vi "[TEST] A3200 Control.vi"() -> ()   [LabVIEW 2026]
uses:
  <extravilib>/ChannelInstances/Tag-str/Write With Abort.vi
  <extravilib>/ChannelInstances/Tag-str/Read With Abort.vi
  <extravilib>/ChannelInstances/Tag-str/Instantiate.vi
  <extravilib>/ChannelInstances/Tag-str/EndpointRead.vi
  <instrlib>/A3200/Motion/AbortSingle.vi
  <instrlib>/A3200/Motion/DisableSingle.vi
  <instrlib>/A3200/Motion/EnableSingle.vi
  <instrlib>/A3200/Motion/FreerunSingle.vi
  <extravilib>/ChannelInstances/Tag-str/Endpoint.vi
  <instrlib>/A3200/Parameters/GetAxisParameterString.vi
  <instrlib>/A3200/Parameters/GetAxisParameterDouble.vi
  <extravilib>/ChannelInstances/Tag-str.lvlib
panel:
  in  "Cluster":T1
  in  "Disable Axis":bool
  in  "ACK ALL":bool
  in  "Enable Axis":bool
  out "Velocity Feedback":string
  out "Position Fbk":string
  out "Numeric":dbl format="%#_13g"
  in  "Stop 3":bool
  in  "Axis Select":i32
  in  "Distance":dbl=1000.0 min=0.0 max=2000.0
  in  "Speed":dbl=5000.0 min=0.0 max=50.0
  out "Status":string
  out "Vel Fbk":dbl
  out "Pos Units":string
  out "Vel Units":string
  in  "Disconnect?":bool
  in  "Stop 2":bool
  out "Axis Selected":string
  in  "Stop":bool
  in  "Go To":bool
  in  "Right":bool
  in  "Left":bool
  out "Encoder X Value":dbl
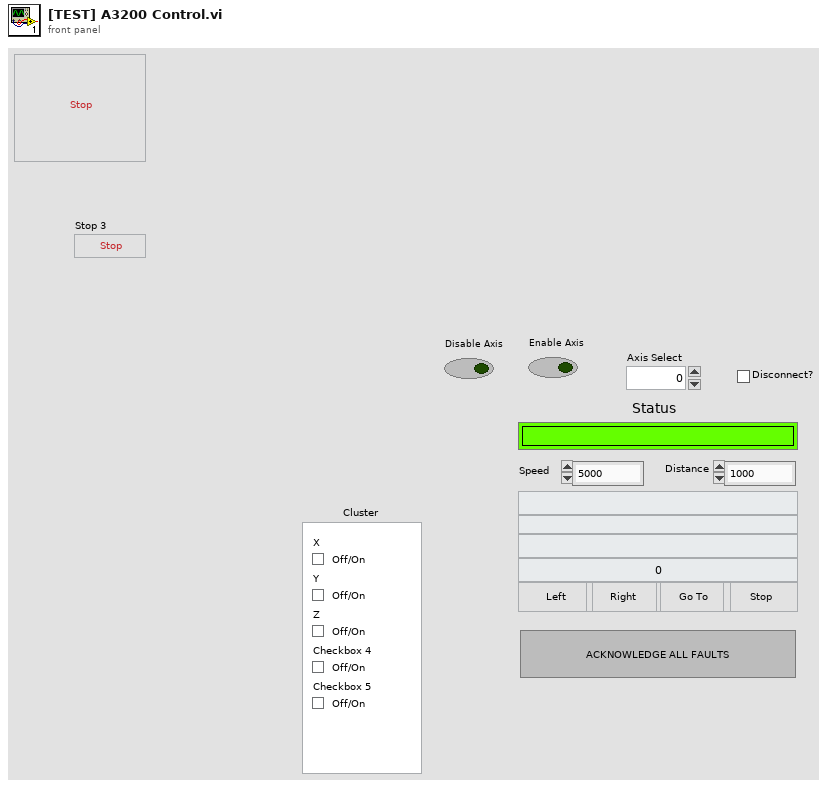
[diagram p1: front panel]
types:
  T1 = cluster{"X":bool, "Y":bool, "Z":bool, "Checkbox 4":bool, "Checkbox 5":bool}
  T2 = cluster{"new reference":refnum<k24>, "Event Callback":refnum<k27>, "ControllerDiagPacket":refnum<user-event>, "Event Registration Refnum":refnum<event-registration>}
  T3 = typedef "AxisDiagPacket.ctl" = cluster{"Axis Name":string, "Analog Input 0":dbl, "Analog Input 1":dbl, "Axis Fault (num)":i32, "Axis Fault (str)":string, "Axis Fault (bits)":cluster{"AmplifierFault":bool, "AmplifierTemperatureFault":bool, "CcwEndOfTravelLimitFault":bool, "CcwSoftwareLimitFault":bool, "CommunicationLostFault":bool, "CwEndOfTravelLimitFault":bool, "CwSoftwareLimitFault":bool, "EmergencyStopFault":bool, "EncoderFault":bool, "ExternalFault":bool, "FeedbackScalingFault":bool, "GantryMisalignFault ":bool, "HallSensorFault":bool, "InPositionTimeoutFault":bool, "MarkerSearchFault":bool, "MaxVelocityCommandFault":bool, "MissedInterruptFault":bool, "MotorTemperatureFault":bool, "None":bool, "OverCurrentFault":bool, "PositionErrorFault":bool, "PositionFeedbackFault":bool, "PowerSupplyFault":bool, "ProbeInputFault":bool, "SafeZoneFault":bool, "VelocityErrorFault":bool, "VelocityFeedbackFault":bool, "VoltageClampFault":bool, "InternalFault":bool}, "Axis Status (num)":i32, "Axis Status (str)":string, "Axis Status (bits)":cluster{"BacklashActive":bool, "CalibrationEnabled1D":bool, "CalibrationEnabled2D":bool, "CommandValid":bool, "DriveAbortPending":bool, "DrivePending":bool, "Enabling":bool, "GainMappingEnabled":bool, "GantryAligned":bool, "GantryRealigning":bool, "Homed":bool, "Homing":bool, "IFOVEnabled":bool, "JogGenerating":bool, "Jogging":bool, "JoystickControl":bool, "MasterSlaveControl":bool, "MotionBlocked":bool, "MotionClamped":bool, "MoveDone":bool, "None":bool, "NotVirtual":bool, "Profiling":bool, "Stability0":bool, "Stability1":bool, "TrajectoryFiltering":bool, "WaitDone":bool}, "Current Command":sgl, "Current Error":sgl, "Current Feedback":sgl, "Digital Inputs":i32, "Digital Outputs":i32, "Drive Status":i32, "Drive Status (str)":string, "Drive Status (bits)":cluster{"AccelerationPhase":bool, "AutofocusActive":bool, "BrakeOutput":bool, "CcwEndOfTravelLimitInput":bool, "CosineEncoderError":bool, "CurrentClamp":bool, "CwEndOfTravelLimitInput":bool, "DecelerationPhase":bool, "DualLoopActive":bool, "EmergencyStopInput":bool, "Enabled":bool, "EncoderClipping":bool, "GalvoCalibrationEnabled":bool, "GalvoPowerCorrection":bool, "HallAInput":bool, "HallBInput":bool, "HallCInput":bool, "HighResolutionMode":bool, "HomeLimitInput":bool, "InPosition":bool, "InPosition2":bool, "MarkerInput":bool, "MarkerLatch":bool, "MoveActive":bool, "NoMotorSupply":bool, "None":bool, "PowerLimiting":bool, "ProgrammingFlash":bool, "ProgrammingMXH":bool, "PSOHaltLatch":bool, "ServoControl":bool, "SineEncoderError":bool}, "Position Feedback Auxiliary":dbl, "Position Command":dbl, "Position Error":dbl, "Position Feedback":dbl, "Program Position Command":dbl, "Program Position Error":dbl, "Program Position Feedback":dbl, "Velocity Command":dbl, "Velocity Error":dbl, "Velocity Feedback":dbl}
  T4 = typedef "Tag-str.lvlib/))Channel.ctl" = refnum<queue>
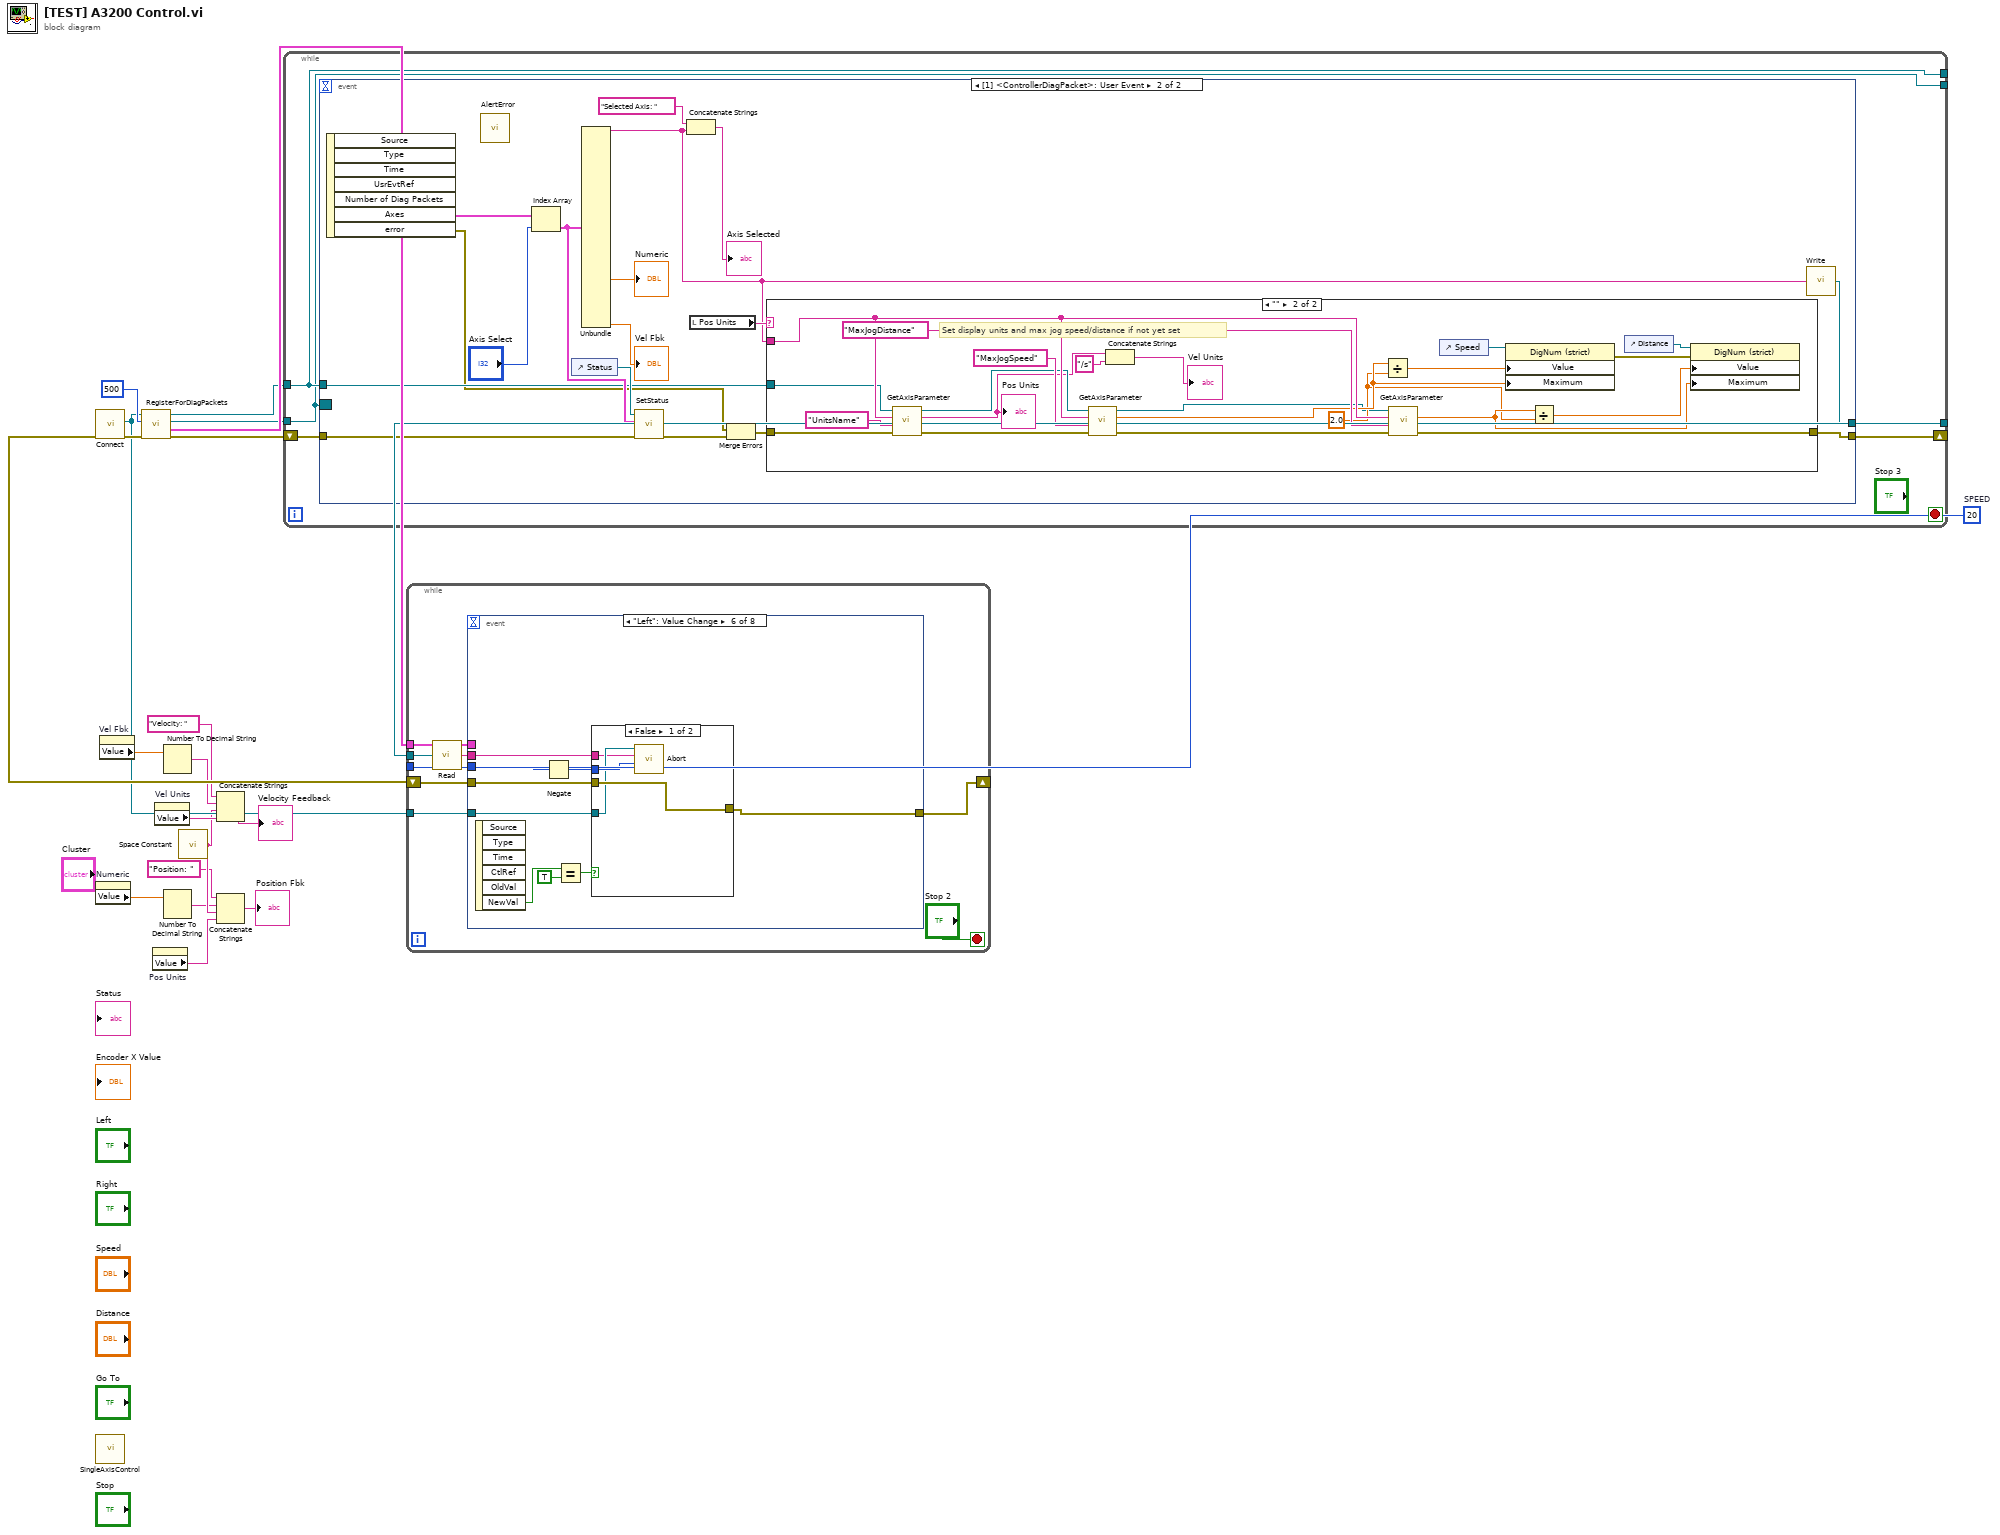
[diagram p0: block diagram]
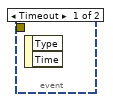
[diagram p2: hidden frame]
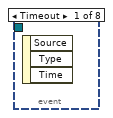
[diagram p4: hidden frame]
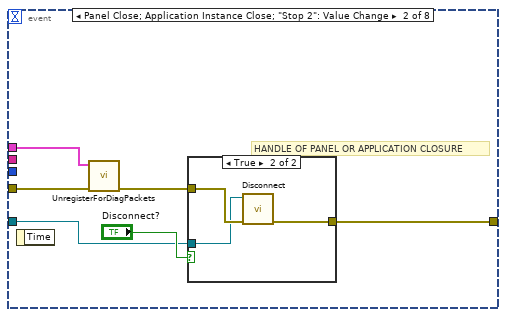
[diagram p5: hidden frame]
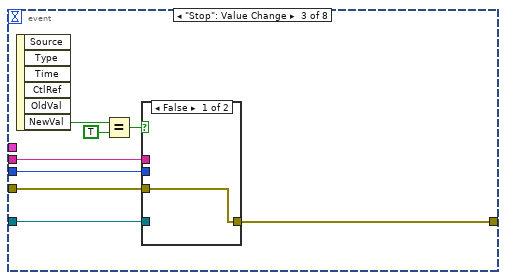
[diagram p7: hidden frame]
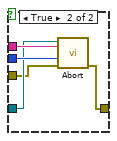
[diagram p8: hidden frame]
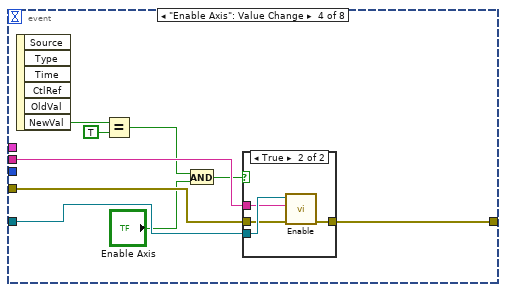
[diagram p9: hidden frame]
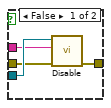
[diagram p10: hidden frame]
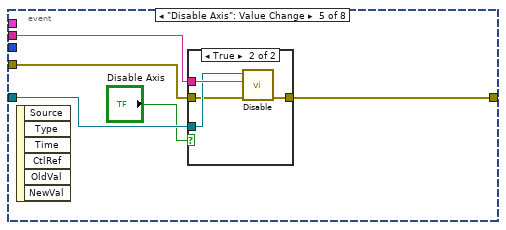
[diagram p11: hidden frame]
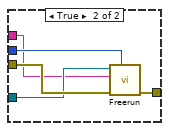
[diagram p13: hidden frame]
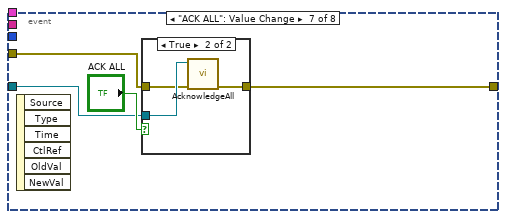
[diagram p14: hidden frame]
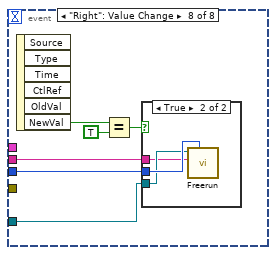
[diagram p16: hidden frame]
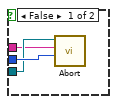
[diagram p17: hidden frame]
diagram:
  w20 = 20  # SPEED
  n1 = call <instrlib>:"Connect.vi"() -> ("error out"=w17:errorcluster, "controller"=w9:refnum<k24>)  [unwired: 10 in]
  n2 = property on="Numeric" class="DigNum (strict)"() -> ("Value"=w13:dbl)  [unwired: 2 in, 2 out]
  n3 = call <instrlib>:"SingleAxisControl.vi"() -> ()  [unwired: 1 in]
  n4 = property on="Vel Fbk" class="DigNum (strict)"() -> ("Value"=w11:dbl)  [unwired: 2 in, 2 out]
  n5 = call <instrlib>:"RegisterForDiagPackets.vi"("error in (no error)"=w17, "refresh interval (default)"=500, "Controller in"=w9) -> ("error out"=w16:errorcluster, "Event Metadata"=w18:T2, "Event Registration Refnum"=w14:refnum<event-registration>, "Controller out"=w15:refnum<k24>)  [unwired: 4 in]
  n6 = property on="Pos Units" class="Str"() -> ("Value"=w4:string)  [unwired: 2 in, 2 out]
  n7 = property on="Vel Units" class="Str"() -> ("Value"=w7:string)  [unwired: 2 in, 2 out]
  n8 = Number To Decimal String(number=w11) -> (decimal integer string=w6:string)  [unwired: 1 in]
  n9 = Number To Decimal String(number=w13) -> (decimal integer string=w2:string)  [unwired: 1 in]
  n10 = call <vilib>:"Space Constant.vi"() -> ("String"=w3:string)
  n11 = Concatenate Strings("Velocity: " ("string"), w6, w3, w7) -> (→"Velocity Feedback":string)
  n12 = Concatenate Strings("Position: " ("string"), w2, w3, w4) -> (→"Position Fbk":string)
  n13 = while {
    shift-right: [w22] -> _
    shift-left: w16 -> [w24]
    tunnel: w15 -> [w26]
    tunnel: [w26] -> _
    tunnel: w14 -> [w23]
    tunnel: [w23] -> _
    tunnel: [w21] -> w8
    stop <- "Stop 3" stop-if-true
    n14 = event shown="[1] <ControllerDiagPacket>: User Event" {
      selector: w23 -> [_ _]
      dyn-events: _ -> [_ _]
      timeout: _ -> [_ _]
      tunnel: w26 -> [_ w37]
      tunnel: w24 -> [_ w36]
      tunnel: [_ w31] -> w22
      tunnel: [_ w30] -> w21
      event Timeout {
        n15 = event-data() -> ()  [unwired: 1 in, 2 out]
      }
      event User Event {
        n16 = event-data() -> ("Axes"=w39:T3[], "error"=w33:errorcluster)  [unwired: 1 in, 5 out]
        n17 = call <instrlib>:"AlertError.vi"() -> ()  [unwired: 11 in, 1 out]
        n18 = Index Array(array=w39, index="Axis Select") -> (element=w41:T3)
        n19 = control-ref of="Status"() -> (w40:refnum<vi>)
        n20 = Unbundle(w41) -> ("Axis Name"=w28:string, "Position Feedback"=→"Numeric":dbl, "Velocity Feedback"=→"Vel Fbk":dbl)  [unwired: 24 out]
        n21 = call <instrlib>:"SetStatus.vi"("error in (no error)"=w36, "AxisDiagPacket"=w41, "Status string"=w40) -> ("error out"=w42:errorcluster)  [unwired: 8 in]
        n22 = Concatenate Strings("Selected Axis: " ("string"), w28) -> (→"Axis Selected":string)
        n23 = local read "Pos Units"() -> (w43:string)
        n24 = Merge Errors(w33, w42) -> (w32:errorcluster)
        n25 = case shown="\"\"" w43 {
          tunnel: w28 -> [_ w61]
          tunnel: w37 -> [_ w48]
          tunnel: w32 -> [w44 w46]
          tunnel: [w44 w45] -> w31
          frame Default {
          }
          frame "" {
            w51 = 2.0 ("y")
            # "Set display units and max jog speed/distance if not yet set"
            n26 = call-poly <instrlib>:"GetAxisParameter.vi"("error in (no error)"=w46, "Parameter Name"="UnitsName" ("parameter name"), "axis name"=w61, "controller in"=w48) -> ("error out"=w62:errorcluster, "value"=w47:string, "controller out"=w49:refnum<k24>)  [unwired: 5 in]
            "Pos Units" <- w47
            n27 = call-poly <instrlib>:"GetAxisParameter.vi"("error in (no error)"=w62, "Parameter Name"="MaxJogSpeed" ("parameter name"), "axis name"=w61, "controller in"=w49) -> ("error out"=w63:errorcluster, "value"=w53:dbl, "controller out"=w50:refnum<k24>)  [unwired: 5 in]
            n28 = Concatenate Strings(w47, "/s" ("string")) -> (→"Vel Units":string)
            n29 = Divide(x=w53, y=w51) -> (x/y=w54:dbl)
            n30 = call-poly <instrlib>:"GetAxisParameter.vi"("error in (no error)"=w63, "Parameter Name"="MaxJogDistance" ("parameter name"), "axis name"=w61, "controller in"=w50) -> ("error out"=w45:errorcluster, "value"=w52:dbl)  [unwired: 5 in, 1 out]
            n31 = control-ref of="Speed"() -> (w58:refnum<vi>)
            n32 = property on="Property Node" class="DigNum (strict)"(reference=w58, "Value"=w54, "Maximum"=w53) -> (error out=w56:errorcluster)  [unwired: 1 in, 1 out]
            n33 = Divide(x=w52, y=w51) -> (x/y=w55:dbl)
            n34 = control-ref of="Distance"() -> (w57:refnum<vi>)
            n35 = property on="Property Node" class="DigNum (strict)"(reference=w57, error in=w56, "Value"=w55, "Maximum"=w52) -> ()  [unwired: 2 out]
          }
        }
        n36 = call <extravilib>:"Write.vi"("element"=w28) -> ("channel"=w30:T4)  [unwired: 1 out]
      }
    }
  }
  n37 = while {
    tunnel: w20 -> [w74]
    tunnel: w18 -> [w72]
    shift-right: [w70] -> _
    shift-left: w16 -> [w71]
    tunnel: w9 -> [w69]
    tunnel: w8 -> [w68]
    stop <- "Stop 2" stop-if-true
    n38 = call <extravilib>:"Read.vi"("channel"=w68) -> ("element"=w67:string)  [unwired: 1 in, 1 out]
    n39 = event shown="[5] \"Left\": Value Change" {
      selector: _ -> [_ _ _ _ _ _ _ _]
      dyn-events: _ -> [_ _ _ _ _ _ _ _]
      timeout: _ -> [_ _ _ _ _ _ _ _]
      tunnel: w74 -> [_ _ w90 _ _ w132 _ w157]
      tunnel: w72 -> [_ w79 _ _ _ _ _ _]
      tunnel: w71 -> [_ w78 w86 w106 w119 w129 w145 _]
      tunnel: [_ w76 w85 w105 w118 w128 w144 _] -> w70
      tunnel: w69 -> [_ w75 w88 w107 w120 w127 w146 w153]
      tunnel: w67 -> [_ _ w87 w104 w117 w126 _ w152]
      event Timeout {
        n40 = event-data() -> ()  [unwired: 1 in, 3 out]
      }
      event Panel Close; Application Instance Close; "Stop 2": Value Change {
        # "HANDLE OF PANEL OR APPLICATION CLOSURE"
        n41 = event-data() -> ()  [unwired: 1 in, 1 out]
        n42 = call <instrlib>:"UnregisterForDiagPackets.vi"("Event Metadata"=w79, "error in (no error)"=w78) -> ("error out"=w77:errorcluster)  [unwired: 8 in]
        n43 = case shown="True" "Disconnect?" {
          tunnel: w77 -> [w81 w84]
          tunnel: [w81 w83] -> w76
          tunnel: w75 -> [_ w82]
          frame False {
          }
          frame True {
            n44 = call <instrlib>:"Disconnect.vi"("error in (no error)"=w84, "controller"=w82) -> ("error out"=w83:errorcluster)  [unwired: 9 in]
          }
        }
      }
      event "Stop": Value Change {
        n45 = event-data() -> ("NewVal"=w92:bool)  [unwired: 1 in, 5 out]
        n46 = Equal?(x=w92, y=TRUE) -> (x = y?=w89:bool)
        n47 = case shown="False" w89 {
          tunnel: w90 -> [_ w97]
          tunnel: w88 -> [_ w96]
          tunnel: w87 -> [_ w98]
          tunnel: w86 -> [w93 w95]
          tunnel: [w93 w94] -> w85
          frame False {
          }
          frame True {
            n48 = call-poly <instrlib>:"Abort.vi"("error in (no error)"=w95, "taskId"=w97, "axis name? (all)"=w98, "controller in"=w96) -> ("error out"=w94:errorcluster)  [unwired: 6 in, 1 out]
          }
        }
      }
      event "Enable Axis": Value Change {
        n49 = event-data() -> ("NewVal"=w103:bool)  [unwired: 1 in, 5 out]
        n50 = Equal?(x=w103, y=TRUE) -> (x = y?=w101:bool)
        n51 = And(x=w101, y="Enable Axis") -> (x .and. y?=w99:bool)
        n52 = case shown="True" w99 {
          tunnel: w107 -> [w111 w115]
          tunnel: w106 -> [w110 w114]
          tunnel: [w109 w113] -> w105
          tunnel: w104 -> [w108 w112]
          frame False {
            n53 = call-poly <instrlib>:"Disable.vi"("error in (no error)"=w110, "axis name"=w108, "controller in"=w111) -> ("error out"=w109:errorcluster)  [unwired: 7 in, 1 out]
          }
          frame True {
            n54 = call-poly <instrlib>:"Enable.vi"("error in (no error)"=w114, "axis name"=w112, "controller in"=w115) -> ("error out"=w113:errorcluster)  [unwired: 7 in, 1 out]
          }
        }
      }
      event "Disable Axis": Value Change {
        n55 = event-data() -> ()  [unwired: 1 in, 6 out]
        n56 = case shown="True" "Disable Axis" {
          tunnel: w120 -> [_ w124]
          tunnel: w119 -> [w121 w123]
          tunnel: [w121 w122] -> w118
          tunnel: w117 -> [_ w125]
          frame False {
          }
          frame True {
            n57 = call-poly <instrlib>:"Disable.vi"("error in (no error)"=w123, "axis name"=w125, "controller in"=w124) -> ("error out"=w122:errorcluster)  [unwired: 7 in, 1 out]
          }
        }
      }
      event "Left": Value Change {
        n58 = event-data() -> ("NewVal"=w134:bool)  [unwired: 1 in, 5 out]
        n59 = Negate(x=w132) -> (-x=w131:i32)
        n60 = Equal?(x=w134, y=TRUE) -> (x = y?=w130:bool)
        n61 = case shown="False" w130 {
          tunnel: w131 -> [w138 w143]
          tunnel: w129 -> [w137 w142]
          tunnel: [w137 w141] -> w128
          tunnel: w127 -> [w136 w140]
          tunnel: w126 -> [w135 w139]
          frame False {
            n62 = call-poly <instrlib>:"Abort.vi"("taskId"=w138, "axis name? (all)"=w135, "controller in"=w136) -> ()  [unwired: 7 in, 2 out]
          }
          frame True {
            n63 = call-poly <instrlib>:"Freerun.vi"("speed"=w143, "error in (no error)"=w142, "axis name"=w139, "controller in"=w140) -> ("error out"=w141:errorcluster)  [unwired: 6 in, 1 out]
          }
        }
      }
      event "ACK ALL": Value Change {
        n64 = event-data() -> ()  [unwired: 1 in, 6 out]
        n65 = case shown="True" "ACK ALL" {
          tunnel: w146 -> [_ w151]
          tunnel: w145 -> [w148 w150]
          tunnel: [w148 w149] -> w144
          frame False {
          }
          frame True {
            n66 = call <instrlib>:"AcknowledgeAll.vi"("error in (no error)"=w150, "controller in"=w151) -> ("error out"=w149:errorcluster)  [unwired: 8 in, 1 out]
          }
        }
      }
      event "Right": Value Change {
        n67 = event-data() -> ("NewVal"=w156:bool)  [unwired: 1 in, 5 out]
        n68 = Equal?(x=w156, y=TRUE) -> (x = y?=w154:bool)
        n69 = case shown="True" w154 {
          tunnel: w157 -> [w160 w163]
          tunnel: w153 -> [w159 w162]
          tunnel: w152 -> [w158 w161]
          frame False {
            n70 = call-poly <instrlib>:"Abort.vi"("taskId"=w160, "axis name? (all)"=w158, "controller in"=w159) -> ()  [unwired: 7 in, 2 out]
          }
          frame True {
            n71 = call-poly <instrlib>:"Freerun.vi"("speed"=w163, "axis name"=w161, "controller in"=w162) -> ()  [unwired: 7 in, 2 out]
          }
        }
      }
    }
  }
